vi "Test String Limit in Report.vi"(11 "Test Case In":refnum<class "Report CSV Content Test.lvclass">) -> (0 "error out":errorcluster, 3 "Test Case Out":refnum<class "Report CSV Content Test.lvclass">)   [LabVIEW 2020, in "Report CSV Content Test.lvclass"]
uses:
  Report CSV Content Test.lvclass
  4993e8ee-a06a-463a-9684-69129f64d5ce.vi
  source/Test Result Handler/TestStand Result Handler.lvclass
  Mock Configuration/Mock Configuration.lvclass
  <vilib>/Astemes/LMock/LMock.lvlib
  <vilib>/Astemes/LMock/One Identical Inputs.vi
  <vilib>/Astemes/LMock/LMock One.lvlib
  C:/Program Files (x86)/National Instruments/LabVIEW 2020/vi.lib/Astemes/LMock/Mock.lvclass
  C:/git/astemes-excel-report-teststand-plugin/tests/Mock Configuration/Mock Configuration.lvclass
  C:/git/astemes-excel-report-teststand-plugin/source/Astemes_CSVReportGenerator/Configuration/Configuration.lvclass
  <vilib>/Astemes/LMock/LMock Verifier.lvclass
  C:/Program Files (x86)/National Instruments/LabVIEW 2020/vi.lib/Astemes/LUnit/Test Case.lvclass
  C:/Program Files (x86)/National Instruments/LabVIEW 2020/vi.lib/Astemes/LUnit/LUnit Runnable.lvclass
  C:/git/astemes-excel-report-teststand-plugin/tests/Test Report CSV Content/Report CSV Content Test.lvclass
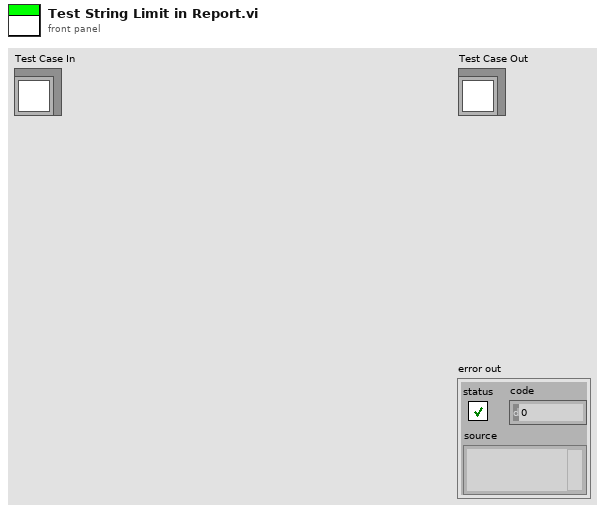
[diagram p1: front panel]
types:
  T1 = typedef "Astemes_CSVReportPlugin.lvlib/TestStand Result Handler.lvclass/TestStand Result.ctl" = cluster{"error in (no error)":errorcluster, "ReportText":string, "TS":cluster{"Index":i32, "BlockLevel":i32, "StartTime":dbl, "Id":i32, "StepType":string, "StepID":string, "StepGroup":string, "StepName":string}, "Status":string}
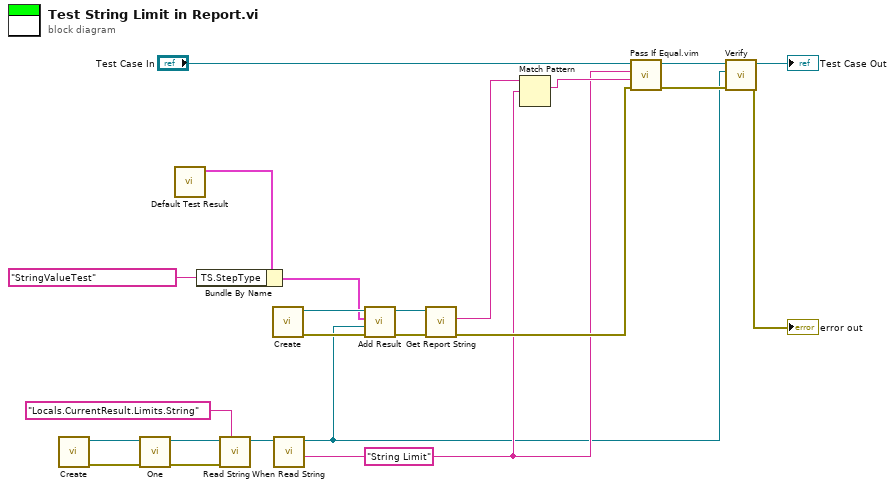
[diagram p0: block diagram]
diagram:
  w5 = "String Limit" ("value")
  n1 = call "Create.vi"() -> ("error out"=w11:errorcluster, "Mock Class Generator out"=w10:refnum<class "Mock Configuration.lvclass">)  [unwired: 10 in]
  n2 = call-poly <vilib>:"One.vi"("error in (no error)"=w11, "Mock in"=w10) -> ("error out"=w8:errorcluster, "Mock out"=w9:refnum<class "Mock Configuration.lvclass">)  [unwired: 8 in]
  n3 = call "Default Test Result.vi"() -> ("TestStand Result"=w17:T1)  [unwired: 11 in]
  n4 = Bundle By Name(cluster=w17, "TS.StepType"="StringValueTest" ("Status")) -> (w16:T1)
  n5 = call-dynamic "Read String.vi"("key"="Locals.CurrentResult.Limits.String", "error in (no error)"=w8, "Configuration In"=w9) -> ("Configuration Out"=w7:refnum<class "Mock Configuration.lvclass">)  [unwired: 6 in, 2 out]
  n6 = call "Create.vi"() -> ("error out"=w20:errorcluster, "Test Result Handler"=w21:refnum<class "TestStand Result Handler.lvclass">)  [unwired: 10 in]
  n7 = call "When Read String.vi"("value"=w5, "Configuration In"=w7) -> ("Configuration Out"=w1:refnum<class "Mock Configuration.lvclass">)  [unwired: 9 in]
  n8 = call "Add Result.vi"("error in (no error)"=w20, "Sequenc Context"=w1, "TestStand Result"=w16, "TestStand Result Handler In"=w21) -> ("error out"=w18:errorcluster, "TestStand Result Handler Out"=w19:refnum<class "TestStand Result Handler.lvclass">)  [unwired: 6 in]
  n9 = call "Get Report String.vi"("error in (no error)"=w18, "TestStand Result Handler In"=w19) -> ("error out"=w12:errorcluster, "Report Text"=w15:string)  [unwired: 8 in]
  n10 = Match Pattern(string=w15, regular expression=w5) -> (match substring=w14:string)  [unwired: 1 in, 3 out]
  n11 = call "Pass If Equal.vim"("error in (no error)"=w12, "Actual"=w14, "Expected"=w5, "LUnit Test Case In"="Test Case In") -> ("error out"=w22:errorcluster, "LUnit Test Case Out"=w3:refnum<class "Report CSV Content Test.lvclass">)  [unwired: 6 in]
  n12 = call <vilib>:"Verify.vi"("error in (no error)"=w22, "Mock"=w1, "LUnit Test Case In"=w3) -> ("error out"=→"error out":errorcluster, "LUnit Test Case Out"=→"Test Case Out":refnum<class "Report CSV Content Test.lvclass">)  [unwired: 7 in]
